vi "Get Position.vi"(11 "Fruit in":refnum<class "Fruit.lvclass">) -> (2 "Coordinates":T1)   [LabVIEW 2020, in "Fruit.lvclass"]
uses:
  Fruit.lvclass
  Snake/Type Defs/Coordinates.ctl
  Fruit.lvclass/Fruit.ctl
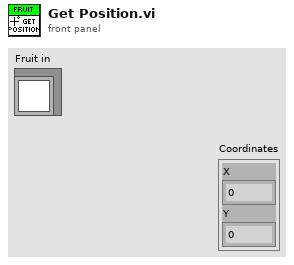
[diagram p1: front panel]
types:
  T1 = typedef "Coordinates.ctl" = cluster{"X":i32, "Y":i32}
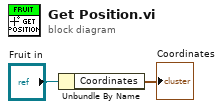
[diagram p0: block diagram]
diagram:
  n1 = Unbundle By Name("Fruit in") -> ("Coordinates"=→"Coordinates":T1)
